vi "sub_logpath.vi"() -> (3 "appended path":path)   [LabVIEW 2018]
uses:
  Global_val.vi
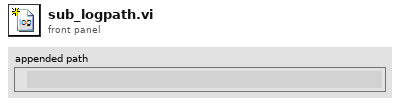
[diagram p1: front panel]
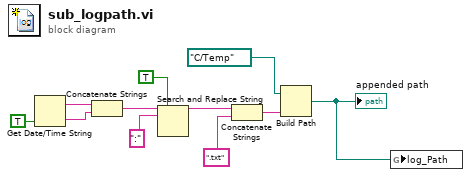
[diagram p0: block diagram]
diagram:
  n1 = Get Date/Time String(want seconds? (F)=TRUE) -> (date string=w4:string, time string=w3:string)  [unwired: 2 in]
  n2 = Concatenate Strings(w4, w3) -> (w5:string)
  n3 = Search and Replace String(replace all?=TRUE ("replace all? (F)"), input string=w5, search string=":") -> (result string=w8:string)  [unwired: 5 in, 3 out]
  n4 = Concatenate Strings(w8, ".txt" ("string")) -> (w10:string)
  n5 = Build Path(base path=path "C:/Temp" ("dup path"), name or relative path=w10) -> (appended path=w1:path)
  "appended path" <- w1
  n6 = global write "Global_val.vi" "log_Path"(w1) -> ()
